vi "DAQInfo Save.vi"(4 "EXP Note":string, 5 "Total time":sgl, 6 "Aline Rate":i32, 7 "# Image Rpt":i32=1, 8 "Y mm":sgl, 9 "X mm":sgl, 10 "Save Name":string="SpctRaw", 11 "Save Path":path=path "D:/OCT Imaging/EXPERIMENT") -> ()   [LabVIEW 2017]
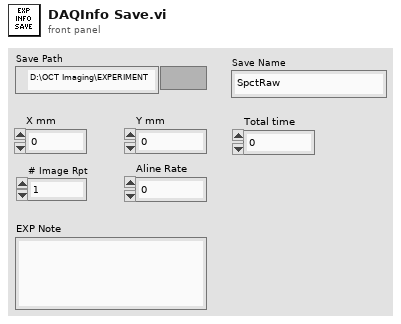
[diagram p1: front panel]
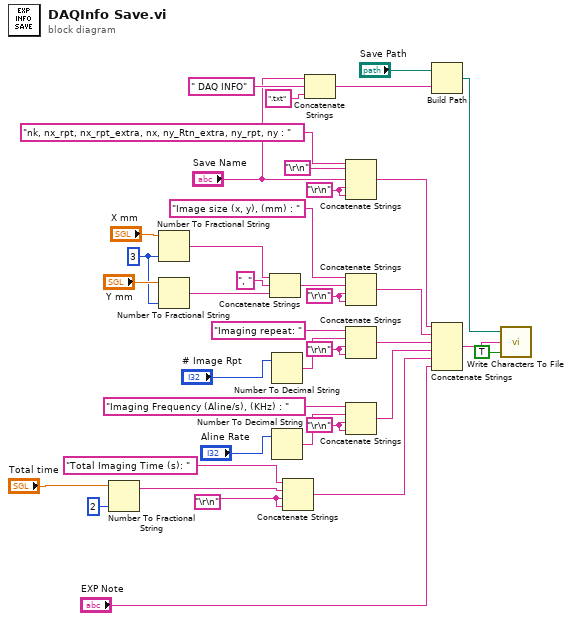
[diagram p0: block diagram]
diagram:
  w8 = "\r\n"
  w10 = i16 3 ("precision (6)")
  w27 = "\r\n"
  w28 = "\r\n"
  w34 = "\r\n"
  w36 = "\r\n"
  n1 = Number To Fractional String(number="Total time", precision (6)=i16 2) -> (F-format string=w7:string)  [unwired: 2 in]
  n2 = Number To Fractional String(number="X mm", precision (6)=w10) -> (F-format string=w15:string)  [unwired: 2 in]
  n3 = Number To Fractional String(number="Y mm", precision (6)=w10) -> (F-format string=w13:string)  [unwired: 2 in]
  n4 = Concatenate Strings(w15, ", " ("string"), w13) -> (w33:string)
  n5 = Number To Decimal String(number="# Image Rpt") -> (decimal integer string=w29:string)  [unwired: 1 in]
  n6 = Number To Decimal String(number="Aline Rate") -> (decimal integer string=w18:string)  [unwired: 1 in]
  n7 = Concatenate Strings("Total Imaging Time (s): " ("string"), w7, w8, w8) -> (w5:string)
  n8 = Concatenate Strings("Save Name", " DAQ INFO" ("string"), ".txt" ("string")) -> (w39:string)
  n9 = Concatenate Strings("nk, nx_rpt, nx_rpt_extra, nx, ny_Rtn_extra, ny_rpt, ny : " ("string"), "\r\n", "Save Name", w34, w34) -> (w26:string)
  n10 = Concatenate Strings("Image size (x, y), (mm) : " ("string"), w33, w28, w28) -> (w25:string)
  n11 = Concatenate Strings("Imaging repeat: " ("string"), w29, w27, w27) -> (w24:string)
  n12 = Concatenate Strings("Imaging Frequency (Aline/s), (KHz) : " ("string"), w18, w36, w36) -> (w23:string)
  n13 = Build Path(base path="Save Path", name or relative path=w39) -> (appended path=w21:path)
  n14 = Concatenate Strings(w26, w25, w24, w23, w5, "EXP Note") -> (w22:string)
  n15 = call <vilib>:"Write Characters To File.vi"("append to file? (new file:F)"=TRUE, "character string"=w22, "file path (dialog if empty)"=w21) -> ()  [unwired: 2 in, 1 out]
